vi "Mysql data reader 1D I64.vi"(8 "error in (no error)":errorcluster, 11 ".NET Refnum in":refnum<k24>) -> (0 "error out":errorcluster, 3 "Array":i64[](array[numeric]))   [LabVIEW 2020, in "mysql.lvlib" / "mysql.lvclass"]
uses:
  mysql.lvclass
  MySql.Data
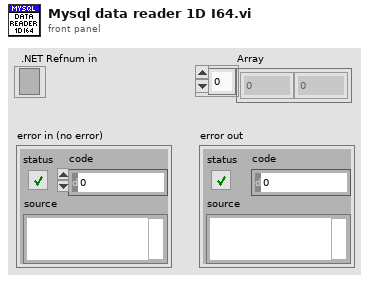
[diagram p1: front panel]
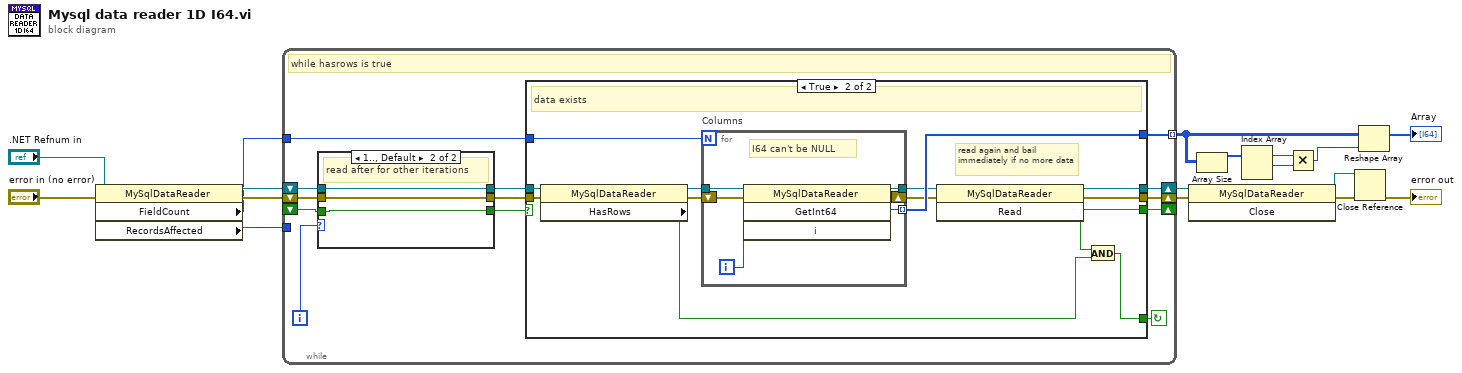
[diagram p0: block diagram]
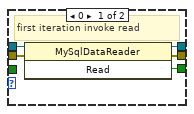
[diagram p2: hidden frame]
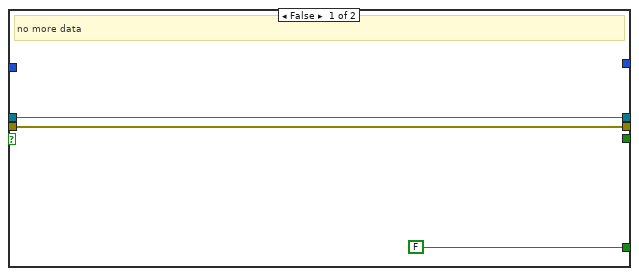
[diagram p3: hidden frame]
diagram:
  n1 = property class="MySqlDataReader"(reference=".NET Refnum in", error in="error in (no error)") -> (reference out=w12:refnum<k24>, error out=w11:errorcluster, "FieldCount"=w9:i32, "RecordsAffected"=w17:i32)
  n2 = while {
    tunnel: w9 -> [w30]
    tunnel: [w29] -> w5 mode=indexing
    shift-right: [w27] -> w14
    shift-left: w11 -> [w24]
    shift-right: [w28] -> w13
    shift-left: w12 -> [w25]
    tunnel: w17 -> [_]
    shift-right: [w20] -> _
    shift-left: _ -> [w18]
    i -> [w19]
    stop <- w26 continue-if-true
    # "while hasrows is true"
    n3 = case shown="1.., Default" w19 {
      tunnel: w24 -> [w35 w37]
      tunnel: [w34 w37] -> w22
      tunnel: w25 -> [w33 w38]
      tunnel: [w32 w38] -> w23
      tunnel: [w31 w36] -> w21
      tunnel: w18 -> [_ w36]
      frame 0 {
        # "first iteration invoke read"
        n4 = invoke class="MySqlDataReader" method="Read"(reference=w33, error in=w35) -> (reference out=w32:refnum<k24>, error out=w34:errorcluster, "Read"=w31:bool)  [unwired: 1 in]
      }
      frame 1.., Default {
        # "read after for other iterations"
      }
    }
    n5 = case shown="True" w21 {
      tunnel: w30 -> [_ w54]
      tunnel: [_ w53] -> w29
      tunnel: w22 -> [w40 w52]
      tunnel: w23 -> [w41 w51]
      tunnel: [w41 w46] -> w28
      tunnel: [w40 w45] -> w27
      tunnel: [FALSE ("HasRows") w42] -> w26
      tunnel: [_ w44] -> w20
      frame False {
        # "no more data"
      }
      frame True {
        # "read again and bail immediately if no more data"
        # "data exists"
        n6 = property class="MySqlDataReader"(reference=w51, error in=w52) -> (reference out=w50:refnum<k24>, error out=w49:errorcluster, "HasRows"=w43:bool)
        n7 = for "Columns" {
          N: w54 -> [_]
          tunnel: w50 -> [w55]
          shift-right: [w60] -> w47
          shift-left: w49 -> [w56]
          tunnel: [w59] -> w53 mode=indexing
          tunnel: [w58] -> w48
          i -> [w57]
          # "I64 can't be NULL"
          n8 = invoke class="MySqlDataReader" method="GetInt64"(reference=w55, error in=w56, "i"=w57) -> (reference out=w58:refnum<k24>, error out=w60:errorcluster, "GetInt64"=w59:i64)  [unwired: 1 in, 1 out]
        }
        n9 = invoke class="MySqlDataReader" method="Read"(reference=w48, error in=w47) -> (reference out=w46:refnum<k24>, error out=w45:errorcluster, "Read"=w44:bool)  [unwired: 1 in]
        n10 = And(x=w44, y=w43) -> (x .and. y?=w42:bool)
      }
    }
  }
  n11 = invoke class="MySqlDataReader" method="Close"(reference=w13, error in=w14) -> (reference out=w16:refnum<k24>, error out=w15:errorcluster)  [unwired: 1 in, 1 out]
  n12 = Array Size(array=w5) -> (size(s)=w6:i32[])
  n13 = Index Array(array=w6) -> (element #1=w3:i32, element #2=w2:i32)  [unwired: 2 in]
  n14 = Multiply(x=w3, y=w2) -> (x*y=w1:i32)
  n15 = Close Reference(reference=w16, error in (no error)=w15) -> (error out=→"error out":errorcluster)
  n16 = Reshape Array(w5, w1) -> (→"Array":i64[])
